vi "SizeLimit_checkOnLogfile.vi"(8 "error in":errorcluster, 10 "LV Data":T1={"Numeric Data"=100, "Float Data"=100.123, "String Data"="This is string", "Enum Data"=enum."Enum Item 2", "Array Data"=[1234, 2345, 3456, 4567]}, 11 "Config IN":T2={"TableLogger"=enum."CSV Logger", "DB File Path"=path "C:/LogAnyLVdata/Test.csv", "DB Backup Config"={"Directory"=path "C:/LogAnyLVdata/dBbackup", "UTC Time Format"=FALSE, "On Launch"=TRUE, "Interval (Hours)"=300.0, "Size Multiples (Bytes)"=24}}) -> (0 "error out":errorcluster)   [LabVIEW 2014]
uses:
  TableLogger_Actor/TableLoggerConfig.ctl
  TableLogger_Actor/TableLoggerTypes.ctl
  TableLogger_Actor/TableLoggerBackupConfig.ctl
  TableLogger_Actor/TableLoggerDataCluster.ctl
  TableLogger_Actor/Messages/InsertData_Msg/InsertData Msg.lvclass/InsertData Msg.ctl
  <vilib>/ActorFramework/Message Enqueuer/Message Enqueuer.lvclass/Message Enqueuer.ctl
  <vilib>/ActorFramework/Message Enqueuer/Enqueue.vi
  <vilib>/ActorFramework/Message Priority Queue/Priority Enqueue.vi
  TableLogger_Actor/Messages/InsertData_Msg/InsertData Msg.lvclass
  <vilib>/ActorFramework/Stop Msg/Stop Msg.lvclass
  <vilib>/addons/_JKI Toolkits/Caraya/classes/Test/Test.lvclass
  <vilib>/addons/_JKI Toolkits/Caraya/classes/Assert/Assert.lvclass
  TableLogger_Actor/TableLogger_Actor/TableLogger_Actor.lvclass
  TableLogger_Actor/TableLogger_Actor.lvlib
panel:
  # "Connector Pane"
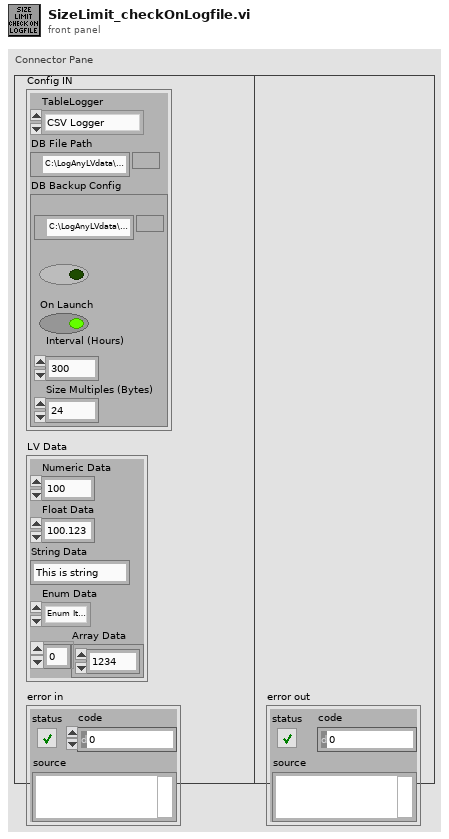
[diagram p1: front panel]
types:
  T1 = typedef "TableLogger_Actor.lvlib/TableLoggerDataCluster.ctl" = cluster{"Numeric Data":i32, "Float Data":dbl, "String Data":string, "Enum Data":enum16{"Enum Item 1", "Enum Item 2"}, "Array Data":i32[]}
  T2 = typedef "TableLogger_Actor.lvlib/TableLoggerConfig.ctl" = cluster{"TableLogger":T3, "DB File Path":path, "DB Backup Config":T4}
  T3 = typedef "TableLogger_Actor.lvlib/TableLoggerTypes.ctl" = enum16{"CSV Logger", "SQLite Logger"}
  T4 = typedef "TableLogger_Actor.lvlib/TableLoggerBackupConfig.ctl" = cluster{"Directory":path, "UTC Time Format":bool, "On Launch":bool, "Interval (Hours)":dbl, "Size Multiples (Bytes)":i32}
  T5 = cluster{"Test Start Timestamp":timestamp, "Test End Timestamp":timestamp, "Test Jig Location":string, "Location Time Offset":string, "Test Jig ID":string, "Test Jig Fluid":enum16{"Liquid", "Gas"}, "Test Jig Flow":enum16{"Low", "High"}, "Control Board SN":string, "Site Number":i32, "Operator ID":string, "Operation Number":string, "DUT Serial Number":string, "DUT Product Number":string, "DUT Flow Range":i32, "DUT FW Revision":string, "DUT TP1 Offset":dbl, "DUT TP2 Offset":dbl, "DUT Cut Off1":dbl, "DUT Cut Off2":dbl, "PreCal Flow Meas":cluster{"FC Flow Set":dbl, "FM Flow Measure":dbl, "UUT Data":dbl}[], "PostCal Flow Meas":cluster{"FC Flow Set":dbl, "FM Flow Measure":dbl, "UUT Data":dbl}[], "DUT_Coeff":dbl[], "DUT_Flow_Error":dbl[], "Calibration Result":enum16{"Pass", "Fail"}}
  T6 = typedef "File Info Record__ogtk.ctl" = cluster{"type":string, "creator":string, "permissions":i32, "data size":i32, "res size":i32, "creation date":u32, "modification date":u32, "bFolder":bool, "bInvisible":bool, "location":cluster{"vertical":i16, "horizontal":i16}, "owner":string, "group":string}
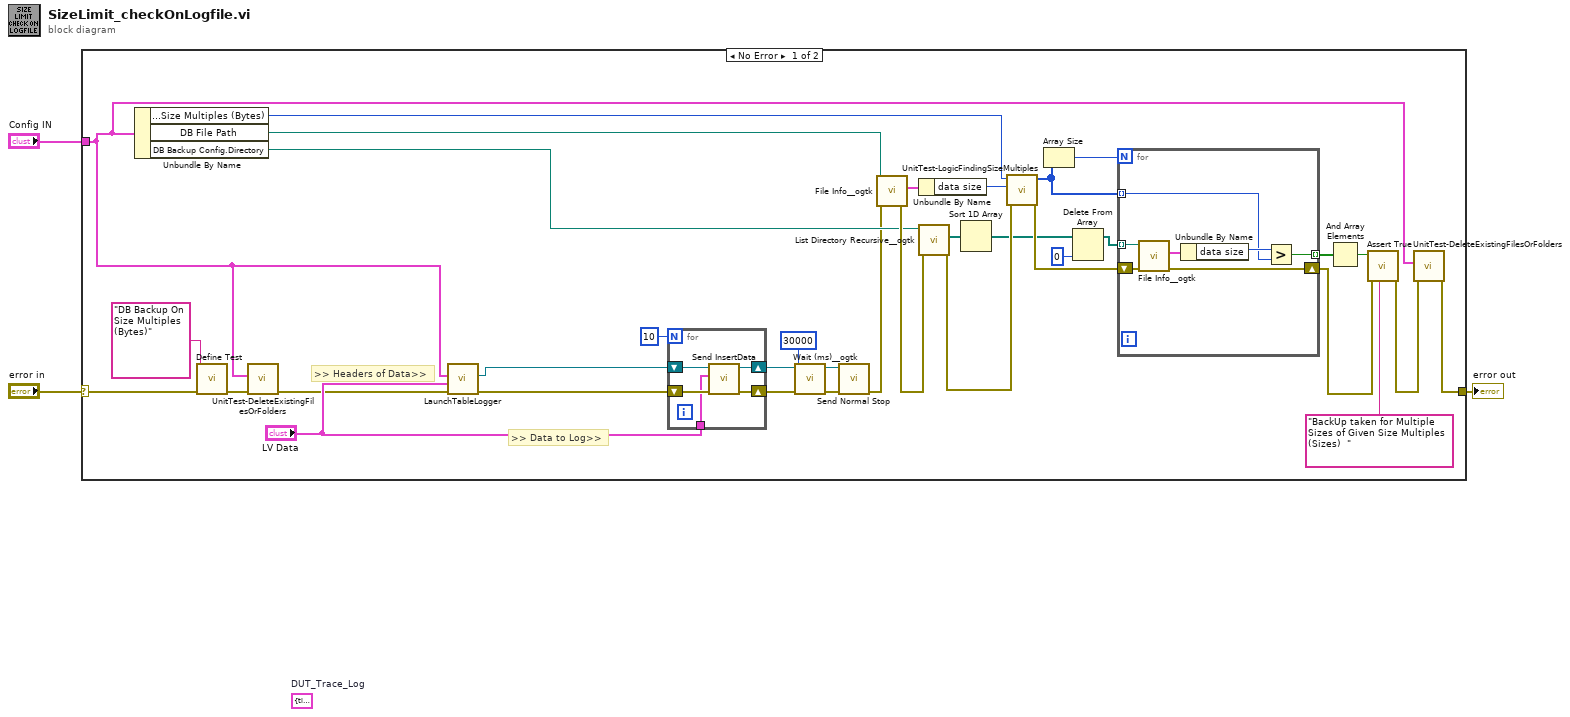
[diagram p0: block diagram]
diagram:
  (unwired) T5 {"Test Start Timestamp"=timestamp(0 s since 1904-01-01), "Test End Timestamp"=timestamp(0 s since 1904-01-01), "Test Jig Location"="asdf", "Location Time Offset"="wer", "Test Jig ID"="xcv", "Test Jig Fluid"=enum."Gas", "Test Jig Flow"=enum."High", "Control Board SN"="fgh", "Site Number"=23, "Operator ID"="op", "Operation Number"="op", "DUT Serial Number"="dt", "DUT Product Number"="dt", "DUT Flow Range"=23, "DUT FW Revision"="asdf", "DUT TP1 Offset"=24.0, "DUT TP2 Offset"=546.0, "DUT Cut Off1"=34.0, "DUT Cut Off2"=453.0, "PreCal Flow Meas"=[{"FC Flow Set"=1.0, "FM Flow Measure"=0.0, "UUT Data"=0.0}, {"FC Flow Set"=2.0, "FM Flow Measure"=0.0, "UUT Data"=0.0}, {"FC Flow Set"=3.0, "FM Flow Measure"=0.0, "UUT Data"=0.0}], "PostCal Flow Meas"=[{"FC Flow Set"=1.0, "FM Flow Measure"=0.0, "UUT Data"=0.0}, {"FC Flow Set"=2.0, "FM Flow Measure"=0.0, "UUT Data"=0.0}], "DUT_Coeff"=[1.0, 2.0], "DUT_Flow_Error"=[1.0, 2.0], "Calibration Result"=enum."Fail"}  # DUT_Trace_Log
  n1 = case shown="No Error" "error in" {
    selector: "error in" -> [w27 w50]
    tunnel: [w17 w50] -> w2
    tunnel: "Config IN" -> [w4 _]
    frame No Error {
      # ">> Headers of Data>>"
      # ">> Data to Log>>"
      n2 = Unbundle By Name(w4) -> ("DB Backup Config.Size Multiples (Bytes)"=w19:i32, "DB File Path"=w16:path, "DB Backup Config.Directory"=w15:path)
      n3 = call <vilib>:"Define Test.vi"("error in (no error)"=w27, "Label (VI Title)"="DB Backup On Size Multiples (Bytes)") -> ("error out"=w26:errorcluster)  [unwired: 9 in]
      n4 = call "UnitTest-DeleteExistingFilesOrFolders.vi"("error in (no error)"=w26, "Config IN"=w4) -> ("error out"=w6:errorcluster)  [unwired: 9 in]
      n5 = call "LaunchTableLogger.vi"("error in (no error)"=w6, "Data Cluster (for Headers)"="LV Data", "TableLogger Config"=w4) -> ("error out"=w13:errorcluster, "TableLogger Actor's Enqueuer"=w14:refnum<class "Message Enqueuer.lvclass">)  [unwired: 5 in, 2 out]
      n6 = for {
        N: 10 -> [_]
        tunnel: "LV Data" -> [w38]
        shift-right: [w39] -> w11
        shift-left: w14 -> [w42]
        shift-right: [w40] -> w12
        shift-left: w13 -> [w41]
        n7 = call "Send InsertData.vi"("error in (no error)"=w41, "Data"=w38, "Message Enqueuer"=w42) -> ("error out"=w40:errorcluster, "Message Enqueuer out"=w39:refnum<class "Message Enqueuer.lvclass">)  [unwired: 7 in]
      }
      n8 = call <userlib>:"Wait (ms)__ogtk.vi"("error in (no error)"=w12, "milliseconds to wait"=u32 30000) -> ("error out"=w9:errorcluster)  [unwired: 8 in, 1 out]
      n9 = call <vilib>:"Send Normal Stop.vi"("error in (no error)"=w9, "Message Enqueuer"=w11) -> ("error out"=w5:errorcluster)  [unwired: 9 in]
      n10 = call <userlib>:"File Info__ogtk.vi"("error in (no error)"=w5, "file"=w16) -> ("error out"=w36:errorcluster, "file info"=w37:T6)  [unwired: 4 in, 1 out]
      n11 = Unbundle By Name(w37) -> ("data size"=w20:i32)
      n12 = call <userlib>:"List Directory Recursive__ogtk.vi"("error in (no error)"=w36, "Path"=w15) -> ("error out"=w33:errorcluster, "file paths"=w34:path[])  [unwired: 6 in, 2 out]
      n13 = Sort 1D Array(array=w34) -> (sorted array=w23:path[])
      n14 = call "UnitTest-LogicFindingSizeMultiples.vi"("error in (no error)"=w33, "File Size"=w20, "DB Multiples Size"=w19) -> ("error out"=w32:errorcluster, "Limits"=w24:i32[])  [unwired: 7 in]
      n15 = Array Size(array=w24) -> (size(s)=w35:i32)
      n16 = Delete From Array(array=w23, index=0) -> (array with subset deleted=w22:path[])  [unwired: 1 in, 1 out]
      n17 = for {
        N: w35 -> [_]
        tunnel: w22 -> [w48] mode=indexing
        shift-right: [w46] -> w29
        shift-left: w32 -> [w47]
        tunnel: [w44] -> w31 mode=indexing
        tunnel: w24 -> [w43] mode=indexing
        n18 = call <userlib>:"File Info__ogtk.vi"("error in (no error)"=w47, "file"=w48) -> ("error out"=w46:errorcluster, "file info"=w49:T6)  [unwired: 4 in, 1 out]
        n19 = Unbundle By Name(w49) -> ("data size"=w45:i32)
        n20 = Greater?(x=w45, y=w43) -> (0:w44:bool)
      }
      n21 = And Array Elements(Boolean array=w31) -> (logical AND=w30:bool)
      n22 = call <vilib>:"Assert True.vi"("Label"="BackUp taken for Multiple Sizes of Given Size Multiples (Sizes)  ", "error in (no error)"=w29, "True?"=w30) -> ("error out"=w18:errorcluster)  [unwired: 8 in]
      n23 = call "UnitTest-DeleteExistingFilesOrFolders.vi"("error in (no error)"=w18, "Config IN"=w4) -> ("error out"=w17:errorcluster)  [unwired: 9 in]
    }
    frame Error {
    }
  }
  "error out" <- w2
